vi "dataconvert_array.vi"(8 "总时间（ms）":dbl, 9 "相乘倍数":i32, 10 "每毫秒采样点":dbl=1.0, 11 "输入的TTL信号序列":dbl[](array[numeric])) -> (2 "输出编码后的TTL序列":dbl[](array[numeric]))   [LabVIEW 2021]
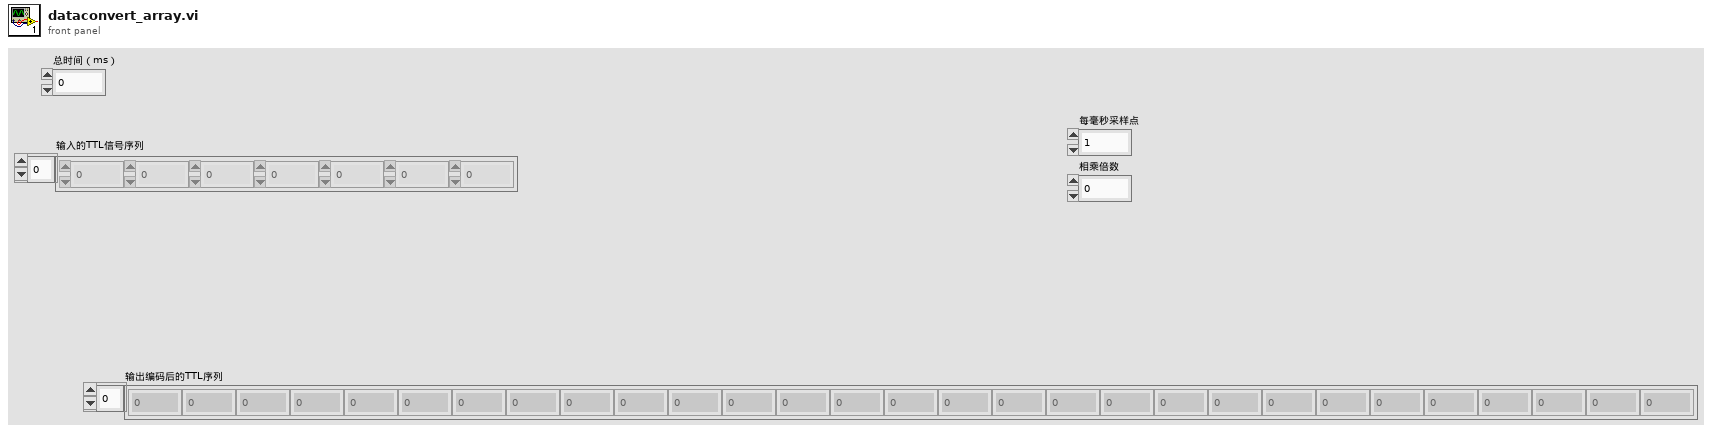
[diagram p1: front panel]
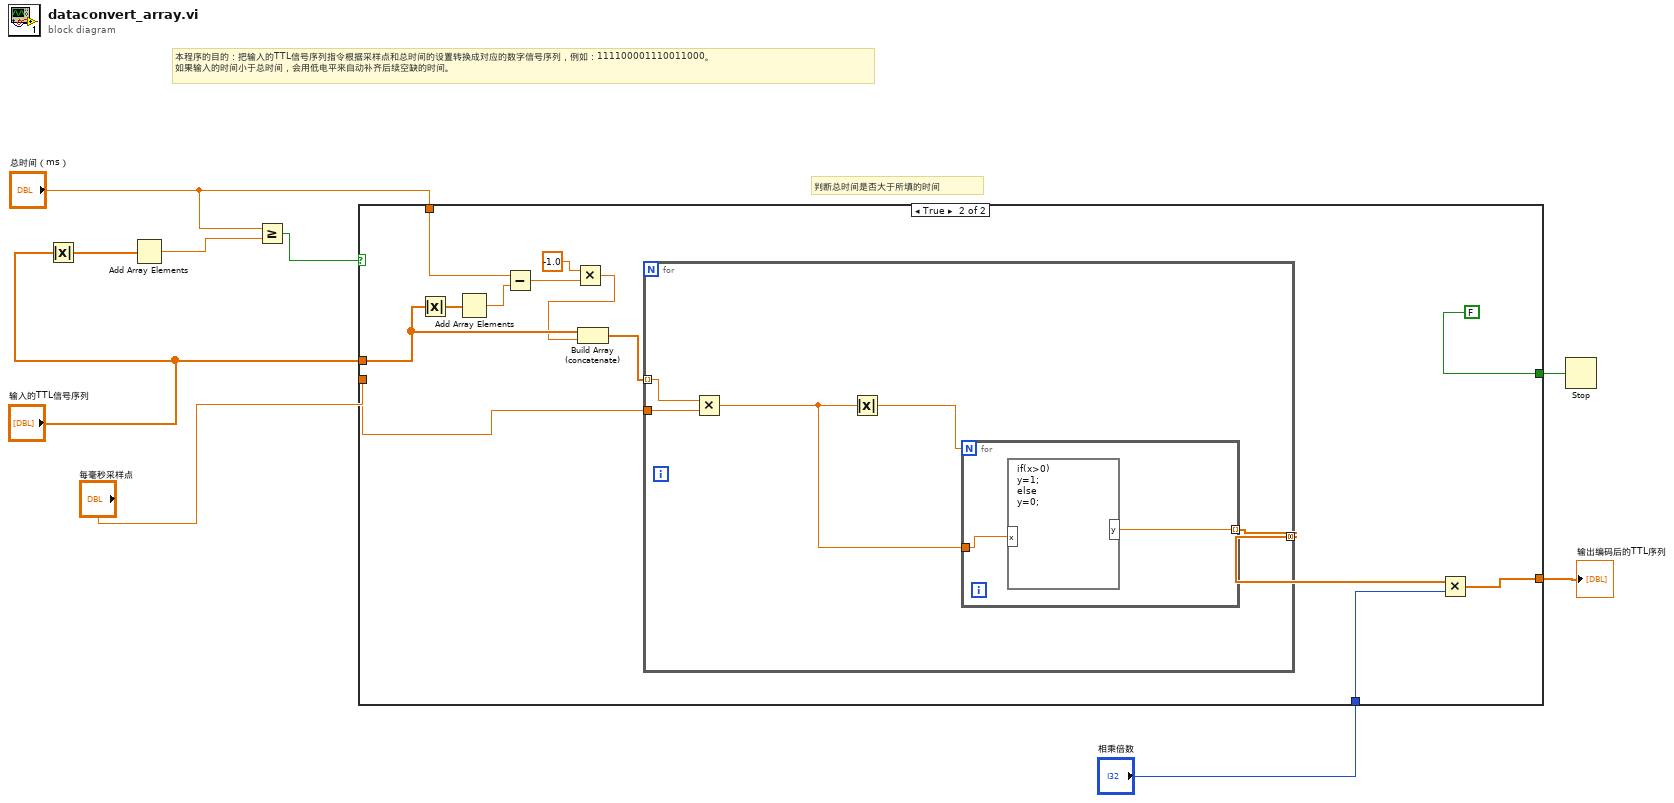
[diagram p0: block diagram]
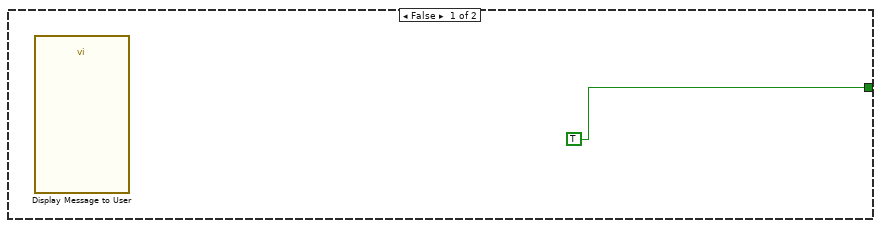
[diagram p2: hidden frame]
diagram:
  # "本程序的目的：把输入的TTL信号序列指令根据采样点和总时间的设置转换成对应的数字信号序列，例如：111100001110011000。\n如果输入的时间小于总时间，会用低电平来自动补齐后续空缺的时间。"
  # "判断总时间是否大于所填的时间"
  n1 = Absolute Value(x="输入的TTL信号序列") -> (abs(x)=w9:dbl[])
  n2 = Add Array Elements(numeric array=w9) -> (sum=w8:dbl)
  n3 = Greater Or Equal?(x="总时间（ms）", y=w8) -> (x >= y?=w7:bool)
  n4 = case shown="True" w7 {
    tunnel: "输入的TTL信号序列" -> [_ w15]
    tunnel: "每毫秒采样点" -> [_ w22]
    tunnel: "相乘倍数" -> [_ w21]
    tunnel: [_ w20] -> w3
    tunnel: [TRUE FALSE] -> w2
    tunnel: "总时间（ms）" -> [_ w16]
    frame False {
      n5 = call "Display Message to User"() -> ()  [unwired: 10 in, 2 out]
    }
    frame True {
      n6 = Absolute Value(x=w15) -> (abs(x)=w18:dbl[])
      n7 = Add Array Elements(numeric array=w18) -> (sum=w17:dbl)
      n8 = Subtract(x=w16, y=w17) -> (x-y=w13:dbl)
      n9 = Multiply(x=-1.0, y=w13) -> (x*y=w11:dbl)
      n10 = Build Array (concatenate)(w15, w11) -> (w14:dbl[])
      n11 = for {
        tunnel: w14 -> [w27] mode=indexing
        tunnel: w22 -> [w28]
        tunnel: [w25] -> w23 mode=concatenating
        n12 = Multiply(x=w27, y=w28) -> (x*y=w24:dbl)
        n13 = Absolute Value(x=w24) -> (abs(x)=w26:dbl)
        n14 = for {
          N: w26 -> [_]
          tunnel: [w30] -> w25 mode=indexing
          tunnel: w24 -> [w29]
          n15 = formula code="if(x>0)\ny=1;\nelse\ny=0;"("x"=w29) -> ("y"=w30:dbl)
        }
      }
      n16 = Multiply(x=w23, y=w21) -> (x*y=w20:dbl[])
    }
  }
  "输出编码后的TTL序列" <- w3
  n17 = Stop(stop? (T)=w2) -> ()
